vi "Tank Fill.vi"() -> ()   [LabVIEW 2013]
uses:
  Tank Fill Global.vi
panel:
  in  "Stop Fill":bool
  in  "Start Fill":bool
  out "Bottom Float Switch":bool
  out "Top Float Switch":bool
  out "Tank level":i32(slide) scale=0.0..300.0
  # "Click          to run"
  # "Tank Fill"
  # "Here, there is a 300 gallon mix tank which mixes red dye.  It drains at a constant rate of 50 gal/sec. There is a pump that can add dye at a rate of 100 gal/sec.\nThere are two float switches, which monitor the level in the tank. When the dye level reaches one of the switches, it is activated, and its value becomes true.\n\nYour job is to add this functionality:\nThe pump is activated by the Start Fill button. When this starts, dye gets pumped into the mix tank until it hits the top float switch. Once this switch is reached, the pump turns off.  \nThe tank level decreases until it the level goes below the bottom float switch. At this point, the pump should start back up and restart the cycle. The tank level should oscillate between the two float switches like this until the stop fill button is pushed, at which point the tank will drain."
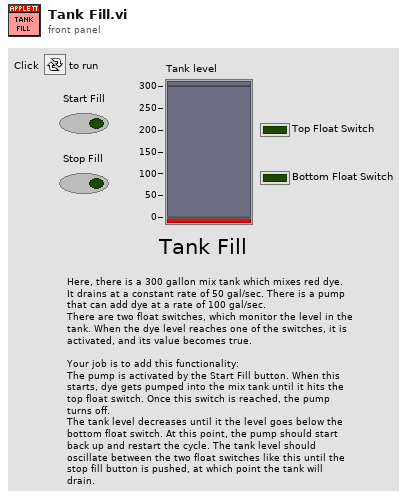
[diagram p1: front panel]
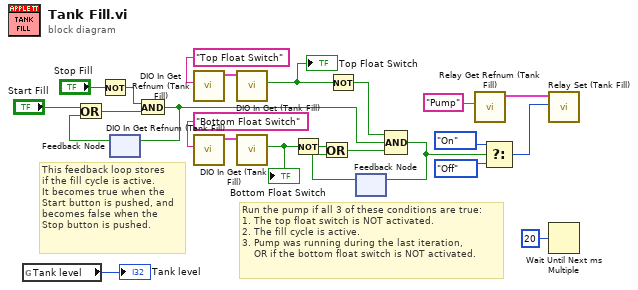
[diagram p0: block diagram]
diagram:
  # "This feedback loop stores\nif the fill cycle is active.\nIt becomes true when the\nStart button is pushed, and\nbecomes false when the \nStop button is pushed."
  # "Run the pump if all 3 of these conditions are true:\n1. The top float switch is NOT activated.\n2. The fill cycle is active.\n3. Pump was running during the last iteration,\n    OR if the bottom float switch is NOT activated."
  n1 = global read "Tank Fill Global.vi" "Tank level"() -> (→"Tank level":i32)
  n2 = Not(x="Stop Fill") -> (.not. x?=w20:bool)
  n3 = feedback #1() -> (w18:bool)  [unwired: 1 in]
  n4 = Or(x="Start Fill", y=w18) -> (x .or. y?=w19:bool)
  n5 = And(x=w20, y=w19) -> (x .and. y?=w10:bool)
  n6 = feedback-in #1(w10) -> ()
  n7 = call "DIO In Get Refnum (Tank Fill).vi"("refnum name"="Top Float Switch") -> ("DigitalInputDevRef"=w13:cluster{string, i32})  [unwired: 9 in, 1 out]
  n8 = call "DIO In Get Refnum (Tank Fill).vi"("refnum name"="Bottom Float Switch") -> ("DigitalInputDevRef"=w17:cluster{string, i32})  [unwired: 9 in, 1 out]
  n9 = call "DIO In Get (Tank Fill).vi"("DigitalInputDevRef"=w13) -> ("Value"=w2:bool)  [unwired: 8 in, 2 out]
  "Top Float Switch" <- w2
  n10 = call "DIO In Get (Tank Fill).vi"("DigitalInputDevRef"=w17) -> ("Value"=w1:bool)  [unwired: 8 in, 2 out]
  "Bottom Float Switch" <- w1
  n11 = Not(x=w1) -> (.not. x?=w15:bool)
  n12 = Not(x=w2) -> (.not. x?=w9:bool)
  n13 = feedback #2() -> (w12:bool)  [unwired: 1 in]
  n14 = Or(x=w15, y=w12) -> (x .or. y?=w11:bool)
  n15 = Compound Arithmetic op=AND(w9, w10, w11) -> (w6:bool)
  n16 = feedback-in #2(w6) -> ()
  n17 = call "Relay Get Refnum (Tank Fill).vi"("refnum name"="Pump") -> ("RelayDevRef"=w8:cluster{string, i32})  [unwired: 9 in, 1 out]
  n18 = Select(t=enum16{"Off", "On"}."On" ("RelayValue"), s=w6, f=enum16{"Off", "On"}."Off" ("RelayValue")) -> (s? t:f=w5:enum16{"Off", "On"})
  n19 = call "Relay Set (Tank Fill).vi"("RelayValue"=w5, "RelayDevRef"=w8) -> ()  [unwired: 8 in, 2 out]
  n20 = Wait Until Next ms Multiple(millisecond multiple=u32 20) -> ()  [unwired: 1 out]
